vi "Set Constant Variables.vi"   [LabVIEW 2012]
uses:
  Robot Global Data.vi
types:
  T1 = cluster{"FVoltConst":dbl, "FVoltConst":dbl, "FVoltConst":dbl}
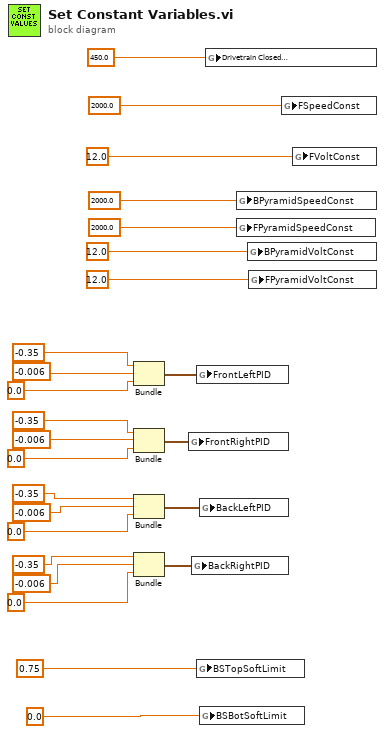
[diagram p0: block diagram]
diagram:
  n1 = Bundle("FVoltConst"=-0.35, "FVoltConst"=-0.006, "FVoltConst"=0.0) -> (w22:T1)  [unwired: 1 in]
  n2 = Bundle("FVoltConst"=-0.35, "FVoltConst"=-0.006, "FVoltConst"=0.0) -> (w20:T1)  [unwired: 1 in]
  n3 = Bundle("FVoltConst"=-0.35, "FVoltConst"=-0.006, "FVoltConst"=0.0) -> (w21:T1)  [unwired: 1 in]
  n4 = Bundle("FVoltConst"=-0.35, "FVoltConst"=-0.006, "FVoltConst"=0.0) -> (w19:T1)  [unwired: 1 in]
  n5 = global write "Robot Global Data.vi" "FrontRightPID"(w20) -> ()
  n6 = global write "Robot Global Data.vi" "BackRightPID"(w19) -> ()
  n7 = global write "Robot Global Data.vi" "FrontLeftPID"(w22) -> ()
  n8 = global write "Robot Global Data.vi" "BSTopSoftLimit"(0.75 ("Drivetrain Closed\nLoop Max")) -> ()
  n9 = global write "Robot Global Data.vi" "BackLeftPID"(w21) -> ()
  n10 = global write "Robot Global Data.vi" "BSBotSoftLimit"(0.0 ("FSpeedConst")) -> ()
  n11 = global write "Robot Global Data.vi" "Drivetrain Closed\nLoop Max"(450.0 ("Drivetrain Closed\nLoop Max")) -> ()
  n12 = global write "Robot Global Data.vi" "BPyramidSpeedConst"(2000.0 ("FSpeedConst")) -> ()
  n13 = global write "Robot Global Data.vi" "FPyramidSpeedConst"(2000.0 ("FSpeedConst")) -> ()
  n14 = global write "Robot Global Data.vi" "BPyramidVoltConst"(12.0 ("FVoltConst")) -> ()
  n15 = global write "Robot Global Data.vi" "FPyramidVoltConst"(12.0 ("FVoltConst")) -> ()
  n16 = global write "Robot Global Data.vi" "FSpeedConst"(2000.0 ("FSpeedConst")) -> ()
  n17 = global write "Robot Global Data.vi" "FVoltConst"(12.0 ("FVoltConst")) -> ()
